vi "Hindbrain_How.vi"(2 "Battery":dbl, 3 "Act Command":cluster{"Velocity":dbl, "Direction":dbl}) -> (1 "HowAmI?":cluster{"T":dbl, "Battery":dbl, "Temp":dbl})   [LabVIEW 2010]
panel:
  # "This sub vi simulates How input by\ndecreasing battery and increasing temperature\nwith respect to speed"
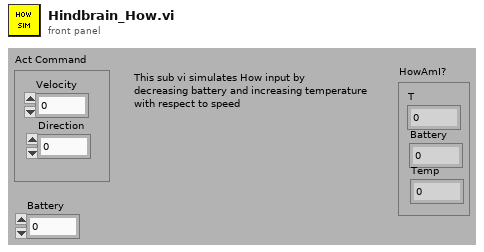
[diagram p1: front panel]
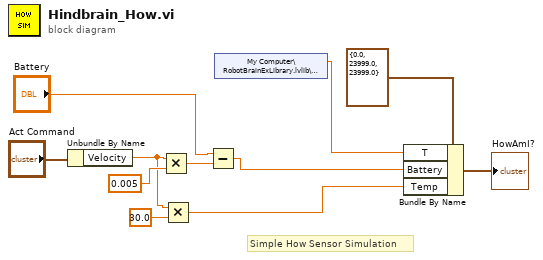
[diagram p0: block diagram]
diagram:
  # "Simple How Sensor Simulation"
  n1 = Unbundle By Name("Act Command") -> ("Velocity"=w3:dbl)
  n2 = Multiply(x=w3, y=0.005) -> (x*y=w6:dbl)
  n3 = Multiply(x=w3, y=30.0) -> (x*y=w1:dbl)
  n4 = Subtract(x="Battery", y=w6) -> (x-y=w4:dbl)
  n5 = shared-variable "My Computer\\RobotBrainExLibrary.lvlib\\MissionTime"() -> (w8:dbl)  [unwired: 1 in, 1 out]
  n6 = Bundle By Name(cluster=cluster{"T":dbl, "Battery":dbl, "Temp":dbl} {"T"=0.0, "Battery"=23999.0, "Temp"=23999.0} ("HowAmI? 2"), "T"=w8, "Battery"=w4, "Temp"=w1) -> (→"HowAmI?":cluster{"T":dbl, "Battery":dbl, "Temp":dbl})
